vi "Teleop.vi"(10 "Match Info":T1={"Autonomous Elapsed Seconds"=0.0, "TeleOp Elapsed Seconds"=0.0, "Disabled Elapsed Seconds"=0.0, "Visited Autonomous"=FALSE, "Visited TeleOp"=FALSE, "Visited Disabled"=FALSE, "Autonomous Settings"={"Autonomous Style"=enum."Independent", "VI Refnum"=refnum}}, 11 "Call Context":T2) -> ()   [LabVIEW 2016]
doc: "This VI is called for each TeleOp packet received from the DS where the robot is not disabled. It is often used to read from the joysticks and update I/O or to update setpoints for timed control loops. It should complete and return within 20 milliseconds or it may miss DS packets."
uses:
  <vilib>/Rock Robotics/WPI/DriverStation/WPI_DriverStationDerivedRobotMode.ctl
  <vilib>/Rock Robotics/WPI/DriverStation/WPI_DriverStationMatch Info.ctl
  <vilib>/Rock Robotics/WPI/Solenoid/WPI_SolenoidValue.ctl
  Robot Global Data.vi
  <vilib>/Rock Robotics/WPI/Utilities/WPI_GetSetVariantRefNum.vi
  <vilib>/Rock Robotics/WPI/Solenoid/Deprecated/WPI_SolenoidSetBool.vi
  <vilib>/Rock Robotics/Network Tables/NT Write Number.vi
  <vilib>/Rock Robotics/Network Tables/NT Write Boolean.vi
  <vilib>/Rock Robotics/WPI/Solenoid/WPI_SolenoidSetEnum.vi
  navX Library v2/navX Library v2.lvlib
panel:
  out "Shooter Values":dbl[](graph)
  out "Shooter Values":cluster{dbl, "Sensor Velocity":dbl, dbl}(graph)
  out "Temperature":dbl(graph)
  in  "Ramp Rate":dbl format="%#_13g"
  in  "I Zone":dbl=3000.0 format="%#_13g"
  in  "F":dbl=0.005212 format="%#_13g"
  in  "D":dbl format="%#_13g"
  in  "I":dbl=0.001 format="%#_13g"
  out "Shooter 2":cluster{"Sensor Velocity":dbl, dbl, dbl}(graph)
  in  "ShooterRPM":dbl=-22000.0
  in  "P":dbl=0.2 format="%#_13g"
  in  "MOE":dbl=25.0 format="%#_13g"
  in  "Center":dbl=180.0 format="%#_13g"
  out "out left":dbl
  out "out right":dbl
  in  "Speed":dbl=0.45 format="%#_13g"
  out "Out Left":dbl(graph)
  out "Out Right":dbl(graph)
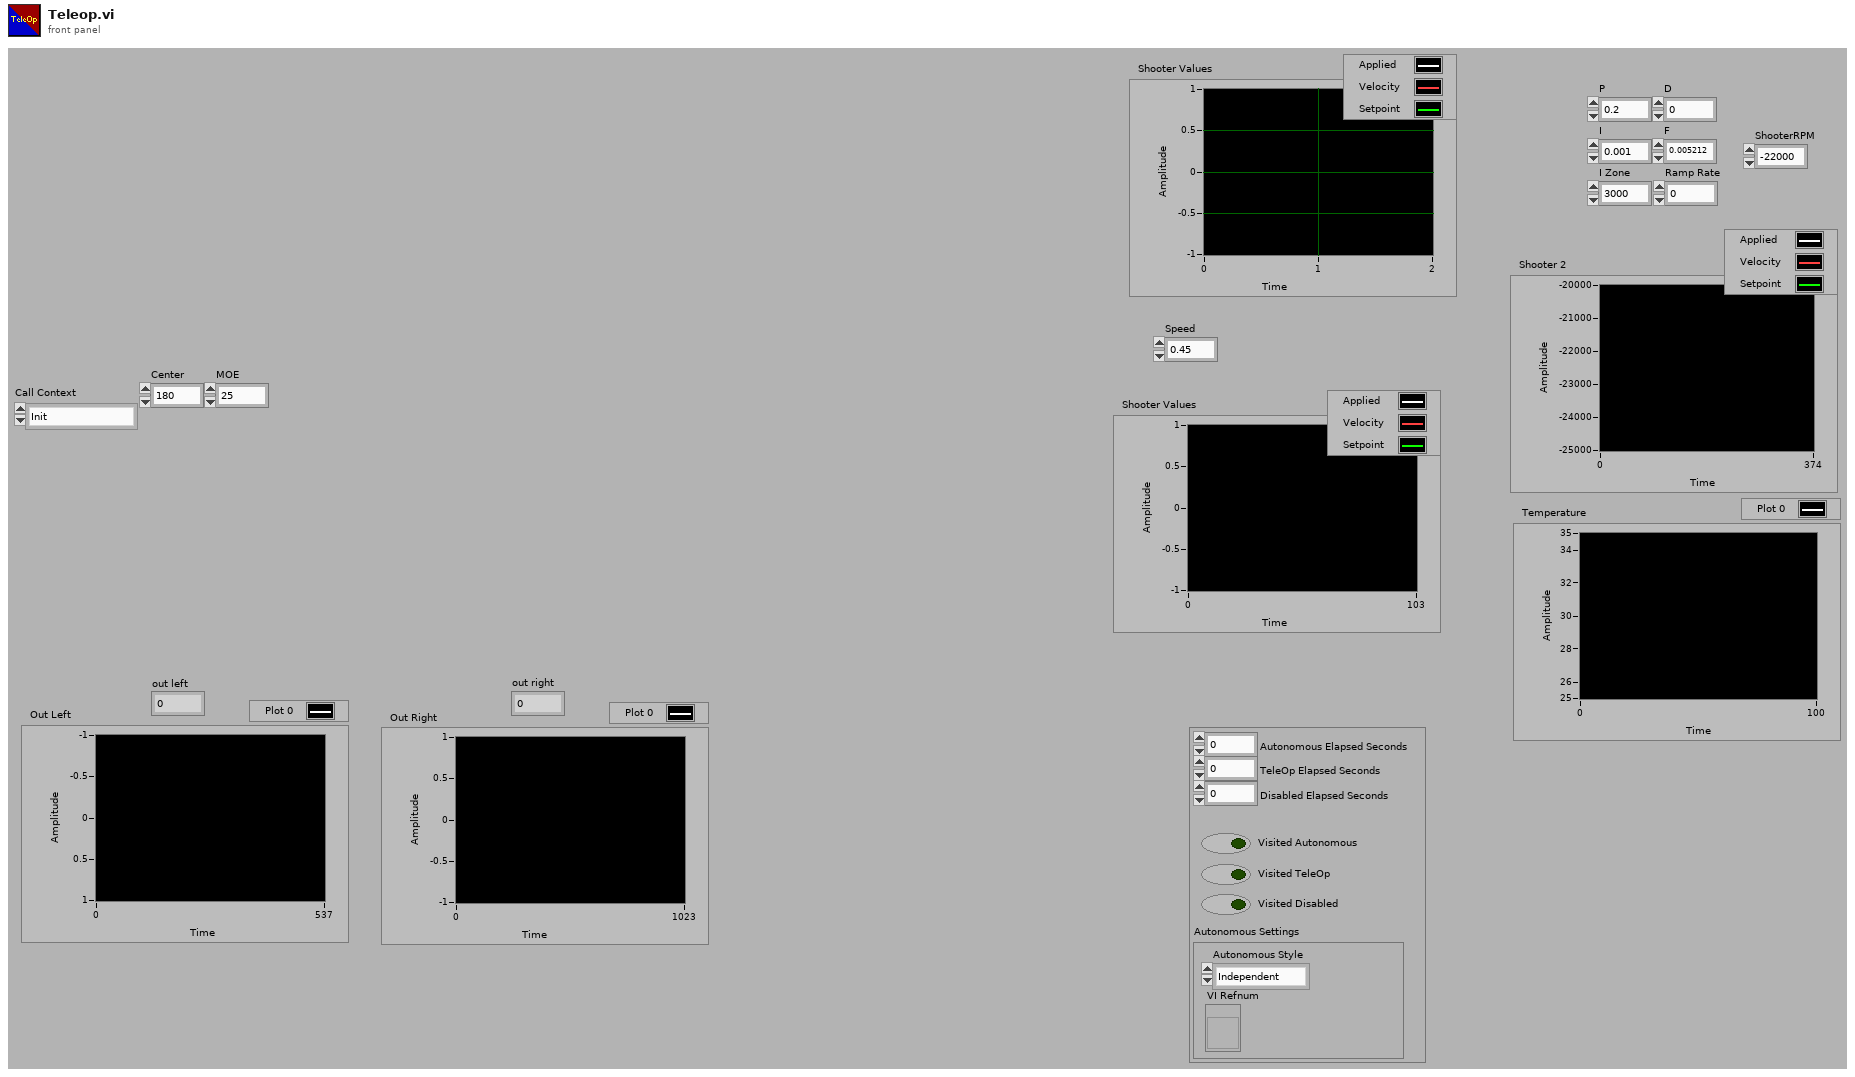
[diagram p1: front panel]
types:
  T1 = typedef "WPI_DriverStationMatch Info.ctl" = cluster{"Autonomous Elapsed Seconds":dbl, "TeleOp Elapsed Seconds":dbl, "Disabled Elapsed Seconds":dbl, "Visited Autonomous":bool, "Visited TeleOp":bool, "Visited Disabled":bool, "Autonomous Settings":cluster{"Autonomous Style":enum16{"Iterative", "Independent"}, "VI Refnum":refnum<vi>}}
  T2 = typedef "WPI_DriverStationDerivedRobotMode.ctl" = enum16{"Init", "Execute", "Stop"}
  T3 = typedef "WPI_SolenoidValue.ctl" = enum16{"Off", "On", "Forward", "Reverse"}
  T4 = typedef "WPI_SolenoidDevRef.ctl" = cluster{"DevStatus":errorcluster, "Pneumatics Control Module":u8, "Forward Solenoid Channel":T5, "Reverse Solenoid Channel":T5}
  T5 = typedef "WPI_SolenoidChannel.ctl" = enum8{"Solenoid 0", "Solenoid 1", "Solenoid 2", "Solenoid 3", "Solenoid 4", "Solenoid 5", "Solenoid 6", "Solenoid 7", "Invalid"}
  T6 = typedef "WPI_JoystickDevRef.ctl" = cluster{"Device":T7}
  T7 = typedef "WPI_JoystickDeviceEnum.ctl" = enum16{"USB 0", "USB 1", "USB 2", "USB 3", "USB 4", "USB 5"}
  T8 = cluster{"Buttons[0]":bool, "Buttons[1]":bool, "Buttons[2]":bool, "Buttons[3]":bool, "Buttons[4]":bool, "Buttons[5]":bool, "Buttons[6]":bool, "Buttons[7]":bool, "Buttons[8]":bool}
  T9 = cluster{"Axes[0]":dbl, "Axes[1]":dbl, "Axes[2]":dbl, "Axes[3]":dbl, "Axes[4]":dbl, "Axes[5]":dbl, "Axes[6]":dbl, "Axes[7]":dbl, "Axes[8]":dbl}
  T10 = typedef "navX Library v2.lvlib/Z900_navX_DeviceTypeDef.ctl" = cluster{"Interface":cluster{"Protocol":T11, "Update Rate (4Hz-100Hz)":u8, "navX Open TypeDef":variant}, "Notify Packet":refnum<notifier>, "Loop VI Refnum":refnum<vi>, "Ready to Close Occurrence Refnum":refnum<k4>}
  T11 = typedef "navX Library v2.lvlib/Z900_navX_ProtocolTypeDef.ctl" = enum16{"SERIAL", "I2C", "SPI"}
  T12 = cluster{"Velocity X":dbl, "Velocity Y":dbl, "Velocity Z":dbl, "Displacement X":dbl, "Displacement Y":dbl, "Displacement Z":dbl}
  T13 = cluster{"LinearAcceleration X":dbl, "LinearAcceleration Y":dbl, "LinearAcceleration Z":dbl}
  T14 = cluster{"Yaw":dbl, "Roll":dbl, "Pitch":dbl, "Heading":dbl, "Fused Heading":dbl}
  T15 = typedef "WPI_MotorControlDeviceRef.ctl" = cluster{"DeviceStatus":errorcluster, "Type":T16, "PWM":cluster{"PWM Channel":T17, "DeadBand":T18}, "CAN":cluster{"Device Number":u8, "SetOutput VI Ref":variant, "GetOutput VI Ref":variant, "Enable VI Ref":variant, "Disable VI Ref":variant, "Data":variant}, "Invert":bool}
  T16 = typedef "WPI_MotorControlType.ctl" = enum16{"PWM", "CAN"}
  T17 = typedef "FPGA_DIOPWMChannel.ctl" = enum8{"PWM 0", "PWM 1", "PWM 2", "PWM 3", "PWM 4", "PWM 5", "PWM 6", "PWM 7", "PWM 8", "PWM 9", "PWM MXP 0", "PWM MXP 1", "PWM MXP 2", "PWM MXP 3", "PWM MXP 4", "PWM MXP 5", "PWM MXP 6", "PWM MXP 7", "PWM MXP 8", "PWM MXP 9", "Invalid"}
  T18 = typedef "WPI_PWMDeadband.ctl" = cluster{"Name":string, "maxPositivePwm":i32, "minPositivePwm":i32, "centerPwm":i32, "maxNegativePwm":i32, "minNegativePwm":i32, "angularRange":u16}
  T19 = typedef "WPI_CANTalonSRX_GlobalStatus.ctl" = cluster{"Applied Throttle":dbl, "Module Enabled":bool, "CAN Error":errorcluster, "Closed Loop Error":dbl, "Forward Limit Switch Closed":bool, "Reverse Limit Switch Closed":bool, "Sensor Position":dbl, "Sensor Velocity":dbl, "Current":dbl, "Sticky Fault - Over Temp":bool, "Sticky Fault - Under Voltage":bool, "Sticky Fault - Forward Limit":bool, "Sticky Fault - Reverse Limit":bool, "Sticky Fault - Forward Soft Limit":bool, "Sticky Fault - Reverse Soft Limit":bool, "Brake is Enabled":bool, "Encoder Position":dbl, "Encoder Velocity":dbl, "Encoder Index Count":dbl, "Encoder A Pin State":bool, "Encoder B Pin State":bool, "Encoder Index Pin State":bool, "Analog In":dbl, "Analog In Velocity":dbl, "Temperature (C)":dbl, "Battery Voltage":dbl, "Control 5 Is Supported":bool, "Current Profile Slot Select":dbl, "Pos Div 8":bool, "Vel Div 4":bool, "Pulse Width Position":i32, "Pulse Width Velocity":i32, "Pulse Width Rise To Rise (us)":i32, "Pulse Width Rise To Fall (us)":i32, "Mot Prof Active Is Under Run":bool, "Mot Prof Active Has Under Run":bool, "Mot Prof Active Is Last":bool, "Mot Prof Active Velocity Only":bool, "Mot Prof Active Is Valid":bool, "Mot Prof Buffer Is Full":bool, "Mot Prof Active Profile Slot Select":i32, "Mot Prof NextID":i32, "Mot Prof Count":i32, "Mot Prof Active Velocity":dbl, "Mot Prof Active Position":dbl, "Mot Prof Output Enable":i32}
  T20 = typedef "WPI_RobotDriveDevRef.ctl" = cluster{"DevStatus":errorcluster, "Motors[]":T15[], "Square Inputs":bool, "Max Output":dbl}
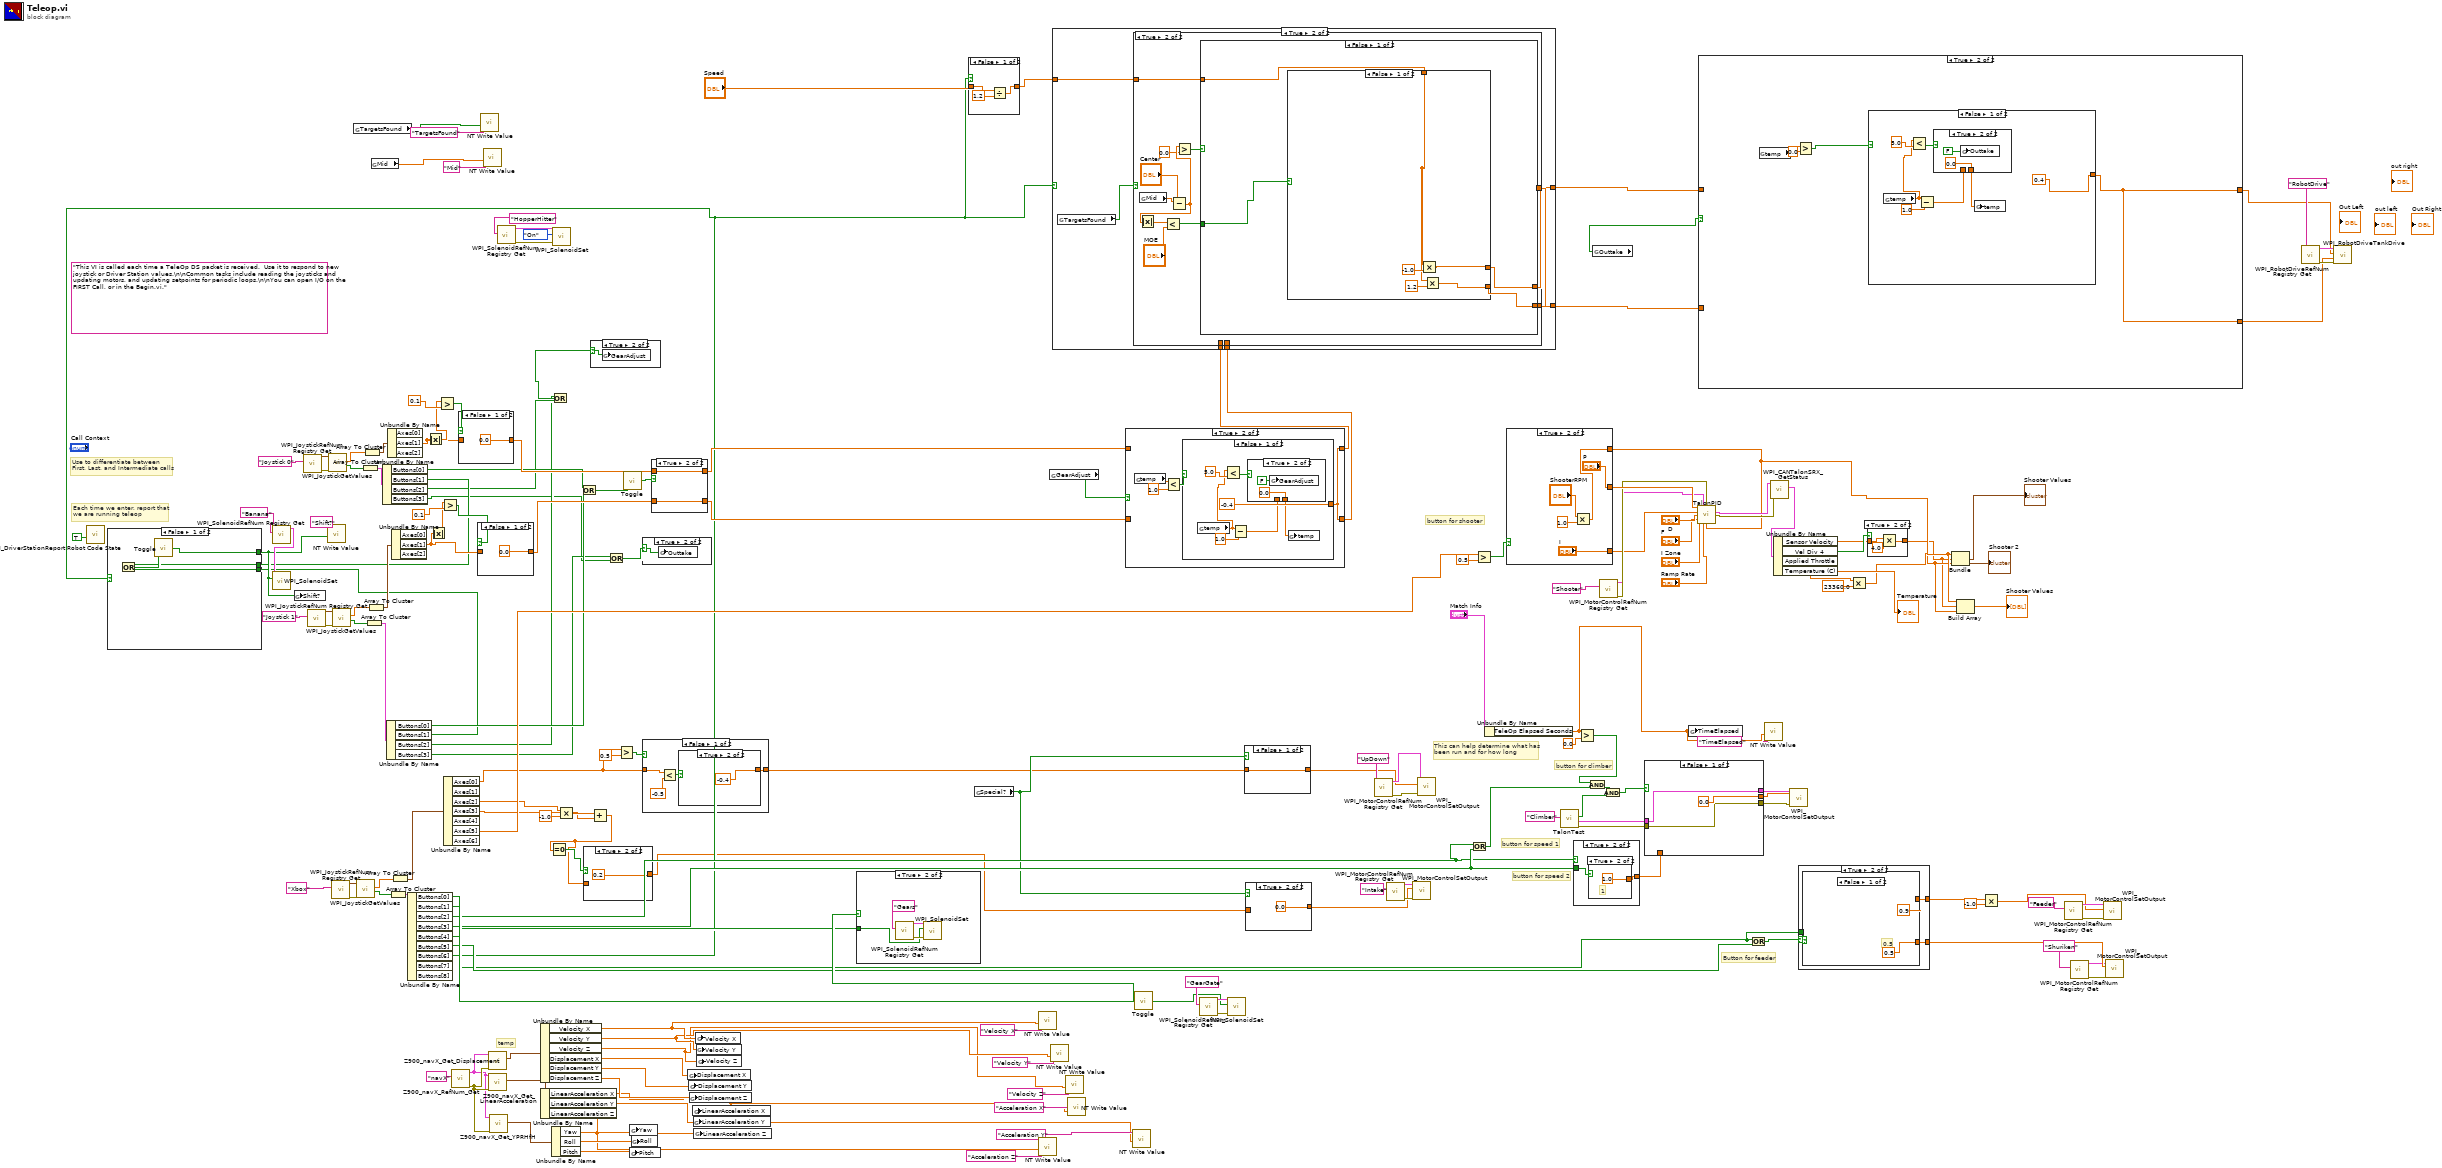
[diagram p0: block diagram]
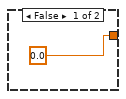
[diagram p3: hidden frame]
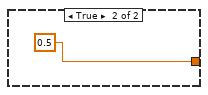
[diagram p4: hidden frame]
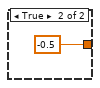
[diagram p6: hidden frame]
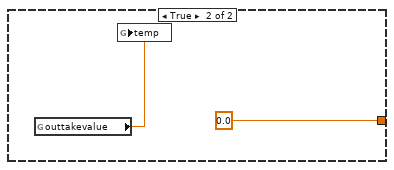
[diagram p9: hidden frame]
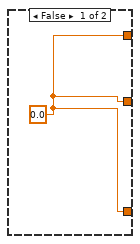
[diagram p12: hidden frame]
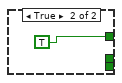
[diagram p13: hidden frame]
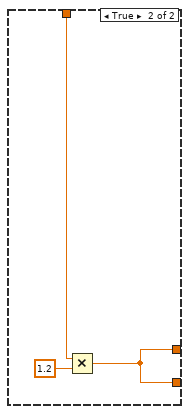
[diagram p17: hidden frame]
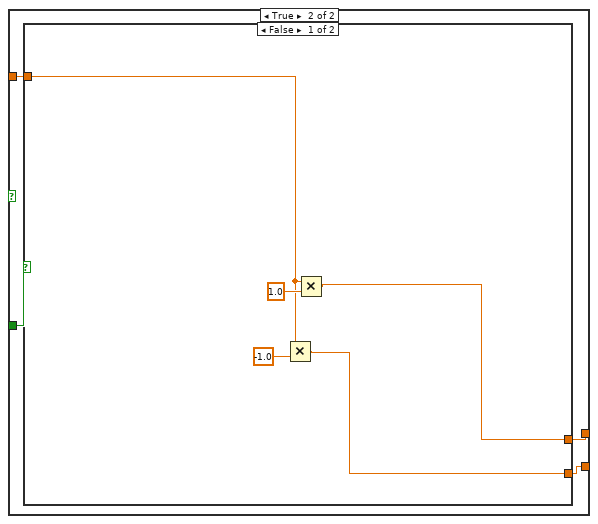
[diagram p18: hidden frame]
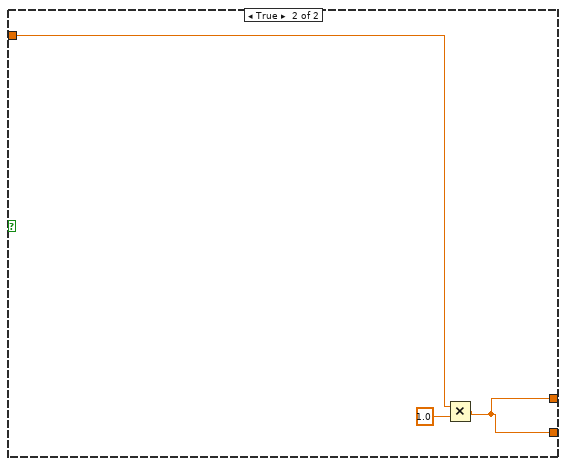
[diagram p19: hidden frame]
diagram:
  (unwired) "This VI is called each time a TeleOp DS packet is received.  Use it to respond to new joystick or Driver Station values.\n\nCommon tasks include reading the joysticks and updating motors, and updating setpoints for periodic loops.\n\nYou can open I/O on the FIRST Call, or in the Begin.vi."
  # "button for shooter"
  # "temp"
  # "Button for feeder"
  # "button for speed 2"
  # "button for speed 1"
  # "button for climber"
  # "Each time we enter, report that\nwe are running teleop"
  # "Use to differentiate between\nFirst, Last, and Intermediate calls"
  # "This can help determine what has\nbeen run and for how long"
  n1 = call <vilib>:"WPI_DriverStationReport Robot Code State.vi"("TeleOp"=TRUE ("Autonomous")) -> ()  [unwired: 10 in, 1 out]
  n2 = call <vilib>:"WPI_SolenoidRefNum Registry Get.vi"("refnum name"="Banana") -> ("SolenoidDevRef"=w94:T4)  [unwired: 9 in, 1 out]
  n3 = call <vilib>:"WPI_JoystickRefNum Registry Get.vi"("refnum name"="Joystick 0") -> ("error out"=w177:errorcluster, "JoystickDevRef"=w176:T6)  [unwired: 9 in]
  n4 = call <vilib>:"WPI_JoystickRefNum Registry Get.vi"("refnum name"="Joystick 1") -> ("error out"=w169:errorcluster, "JoystickDevRef"=w168:T6)  [unwired: 9 in]
  n5 = call <vilib>:"WPI_JoystickGetValues.vi"("error in (no error)"=w177, "JoystickDevRef"=w176) -> ("Buttons"=w173:bool[], "Axes"=w174:dbl[])  [unwired: 5 in, 3 out]
  n6 = call <vilib>:"WPI_JoystickRefNum Registry Get.vi"("refnum name"="Xbox") -> ("error out"=w144:errorcluster, "JoystickDevRef"=w143:T6)  [unwired: 9 in]
  n7 = call <vilib>:"WPI_JoystickGetValues.vi"("error in (no error)"=w169, "JoystickDevRef"=w168) -> ("Buttons"=w165:bool[], "Axes"=w166:dbl[])  [unwired: 5 in, 3 out]
  n8 = global read "Robot Global Data.vi" "TargetsFound"() -> (w98:bool)
  n9 = call <vilib>:"WPI_JoystickGetValues.vi"("error in (no error)"=w144, "JoystickDevRef"=w143) -> ("Buttons"=w140:bool[], "Axes"=w141:dbl[])  [unwired: 5 in, 3 out]
  n10 = Array To Cluster(array=w173) -> (cluster=w171:T8)
  n11 = Array To Cluster(array=w174) -> (cluster=w172:T9)
  n12 = Array To Cluster(array=w165) -> (cluster=w163:T8)
  n13 = Array To Cluster(array=w166) -> (cluster=w164:T9)
  n14 = global read "Robot Global Data.vi" "Mid"() -> (w96:dbl)
  n15 = Unbundle By Name(w171) -> ("Buttons[0]"=w36:bool, "Buttons[1]"=w32:bool, "Buttons[2]"=w31:bool, "Buttons[3]"=w19:bool)
  n16 = Unbundle By Name(w163) -> ("Buttons[0]"=w35:bool, "Buttons[1]"=w33:bool, "Buttons[2]"=w30:bool, "Buttons[3]"=w20:bool)
  n17 = Unbundle By Name(w172) -> ("Axes[1]"=w158:dbl)  [unwired: 2 out]
  n18 = Array To Cluster(array=w140) -> (cluster=w138:T8)
  n19 = Unbundle By Name(w164) -> ("Axes[1]"=w160:dbl)  [unwired: 2 out]
  n20 = Array To Cluster(array=w141) -> (cluster=w139:T9)
  n21 = Unbundle By Name(w138) -> ("Buttons[0]"=w137:bool, "Buttons[1]"=w136:bool, "Buttons[2]"=w37:bool, "Buttons[3]"=w135:bool, "Buttons[4]"=w132:bool, "Buttons[5]"=w133:bool, "Buttons[6]"=w29:bool)  [unwired: 2 out]
  n22 = case shown="False" w29 {
    tunnel: w33 -> [w181 _]
    tunnel: w32 -> [w180 _]
    tunnel: [w179 TRUE] -> w92
    frame False {
      n23 = Or(x=w180, y=w181) -> (x .or. y?=w182:bool)
      n24 = call "Toggle.vi"("Input"=w182) -> ("Output"=w179:bool)
    }
    frame True {
    }
  }
  n25 = call-poly <vilib>:"WPI_SolenoidSet.vi"("Value"=w92, "SolenoidDevRef"=w94) -> ()  [unwired: 8 in, 2 out]
  n26 = global write "Robot Global Data.vi" "Shift?"(w92) -> ()
  n27 = call-poly <vilib>:"NT Write Value.vi"("Boolean"=w92, "Name"="Shift?") -> ()  [unwired: 9 in, 1 out]
  n28 = Absolute Value(x=w158) -> (abs(x)=w159:dbl)
  n29 = Absolute Value(x=w160) -> (abs(x)=w161:dbl)
  n30 = Greater?(x=w159, y=0.1 ("x")) -> (0:w110:bool)
  n31 = Greater?(x=w161, y=0.1 ("x")) -> (0:w109:bool)
  n32 = Unbundle By Name(w139) -> ("Axes[0]"=w5:dbl, "Axes[2]"=w28:dbl, "Axes[3]"=w25:dbl, "Axes[5]"=w74:dbl)  [unwired: 3 out]
  n33 = call "Z900_navX_RefNum_Get.vi"("refnum name"="navX") -> ("error out"=w61:errorcluster, "navX Device"=w60:T10)  [unwired: 9 in]
  n34 = case shown="False" w110 {
    tunnel: w158 -> [_ w185]
    tunnel: [0.0 w185] -> w107
    frame False {
    }
    frame True {
    }
  }
  n35 = case shown="False" w109 {
    tunnel: w160 -> [_ w187]
    tunnel: [0.0 w187] -> w108
    frame False {
    }
    frame True {
    }
  }
  n36 = call-poly <vilib>:"NT Write Value.vi"("Boolean"=w98, "Name"="TargetsFound") -> ()  [unwired: 9 in, 1 out]
  n37 = call-poly <vilib>:"NT Write Value.vi"("Numeric"=w96, "Name"="Mid") -> ()  [unwired: 9 in, 1 out]
  n38 = call "Z900_navX_Get_Displacement.vi"("error in (no error)"=w61, "navX Device"=w60) -> ("Displacement"=w57:T12)  [unwired: 6 in, 3 out]
  n39 = call "Z900_navX_Get_LinearAcceleration.vi"("error in (no error)"=w61, "navX Device"=w60) -> ("Linear Acceleration"=w58:T13)  [unwired: 6 in, 3 out]
  n40 = call "Z900_navX_Get_YPRHfH.vi"("error in (no error)"=w61, "navX Device"=w60) -> ("YRPHfH"=w59:T14)  [unwired: 6 in, 3 out]
  n41 = call <vilib>:"WPI_SolenoidRefNum Registry Get.vi"("refnum name"="HopperHitter") -> ("error out"=w64:errorcluster, "SolenoidDevRef"=w65:T4)  [unwired: 9 in]
  n42 = Unbundle By Name(w57) -> ("Velocity X"=w45:dbl, "Velocity Y"=w44:dbl, "Velocity Z"=w43:dbl, "Displacement X"=w56:dbl, "Displacement Y"=w55:dbl, "Displacement Z"=w54:dbl)
  n43 = Unbundle By Name(w58) -> ("LinearAcceleration X"=w42:dbl, "LinearAcceleration Y"=w39:dbl, "LinearAcceleration Z"=w41:dbl)
  n44 = Or(x=w30, y=w31) -> (x .or. y?=w116:bool)
  n45 = Unbundle By Name(w59) -> ("Yaw"=w53:dbl, "Roll"=w52:dbl, "Pitch"=w51:dbl)
  n46 = call-poly <vilib>:"WPI_SolenoidSet.vi"("error in (no error)"=w64, "Value"=WPI_SolenoidValue."On", "SolenoidDevRef"=w65) -> ()  [unwired: 7 in, 2 out]
  n47 = Multiply(x=w28, y=-1.0) -> (x*y=w26:dbl)
  n48 = Or(x=w36, y=w35) -> (x .or. y?=w34:bool)
  n49 = case shown="True" w116 {
    selector: w116 -> [_ w188]
    frame False {
    }
    frame True {
      n50 = global write "Robot Global Data.vi" "GearAdjust"(w188) -> ()
    }
  }
  n51 = Add(x=w26, y=w25) -> (x+y=w2:dbl)
  n52 = Equal To 0?(x=w2) -> (x = 0?=w3:bool)
  n53 = case shown="True" w3 {
    tunnel: w2 -> [w189 _]
    tunnel: [w189 0.2] -> w1
    frame False {
    }
    frame True {
    }
  }
  n54 = Or(x=w20, y=w19) -> (x .or. y?=w21:bool)
  n55 = Greater?(x=w5, y=0.5) -> (0:w6:bool)
  n56 = call "Toggle.vi"("Input"=w34) -> ("Output"=w104:bool)
  n57 = global write "Robot Global Data.vi" "Pitch"(w51) -> ()
  n58 = global write "Robot Global Data.vi" "Yaw"(w53) -> ()
  n59 = global write "Robot Global Data.vi" "Roll"(w52) -> ()
  n60 = case shown="True" w21 {
    selector: w21 -> [_ w191]
    frame False {
    }
    frame True {
      n61 = global write "Robot Global Data.vi" "Outtake"(w191) -> ()
    }
  }
  n62 = case shown="False" w6 {
    tunnel: w5 -> [w194 _]
    tunnel: [w192 0.5] -> w4
    frame False {
      n63 = Less?(x=w194, y=-0.5) -> (x < y?=w195:bool)
      n64 = case shown="True" w195 {
        tunnel: [0.0 -0.4] -> w192
        frame False {
        }
        frame True {
        }
      }
    }
    frame True {
    }
  }
  n65 = case shown="True" w104 {
    tunnel: w107 -> [w200 w205]
    tunnel: w108 -> [w199 w204]
    tunnel: [w203 w205] -> w106
    tunnel: [w202 w204] -> w105
    frame False {
      w201 = -1.0
      n66 = Multiply(x=w201, y=w200) -> (x*y=w202:dbl)
      n67 = Multiply(x=w199, y=w201) -> (x*y=w203:dbl)
    }
    frame True {
    }
  }
  n68 = global write "Robot Global Data.vi" "Displacement X"(w56) -> ()
  n69 = global write "Robot Global Data.vi" "Displacement Y"(w55) -> ()
  n70 = global write "Robot Global Data.vi" "Displacement Z"(w54) -> ()
  n71 = global write "Robot Global Data.vi" "LinearAcceleration X"(w42) -> ()
  n72 = global write "Robot Global Data.vi" "LinearAcceleration Y"(w39) -> ()
  n73 = global write "Robot Global Data.vi" "LinearAcceleration Z"(w41) -> ()
  n74 = global write "Robot Global Data.vi" "Velocity X"(w45) -> ()
  n75 = global write "Robot Global Data.vi" "Velocity Y"(w44) -> ()
  n76 = global write "Robot Global Data.vi" "Velocity Z"(w43) -> ()
  n77 = case shown="False" w29 {
    tunnel: [w208 w209] -> w102
    tunnel: "Speed" -> [w207 w209]
    frame False {
      n78 = Divide(x=w207, y=1.2) -> (x/y=w208:dbl)
    }
    frame True {
    }
  }
  n79 = global read "Robot Global Data.vi" "Special?"() -> (w12:bool)
  n80 = call-poly <vilib>:"NT Write Value.vi"("Numeric"=w45, "Name"="Velocity X") -> ()  [unwired: 9 in, 1 out]
  n81 = call-poly <vilib>:"NT Write Value.vi"("Numeric"=w41, "Name"="Acceleration Z") -> ()  [unwired: 9 in, 1 out]
  n82 = global read "Robot Global Data.vi" "GearAdjust"() -> (w117:bool)
  n83 = call-poly <vilib>:"NT Write Value.vi"("Numeric"=w44, "Name"="Velocity Y") -> ()  [unwired: 9 in, 1 out]
  n84 = call-poly <vilib>:"NT Write Value.vi"("Numeric"=w43, "Name"="Velocity Z") -> ()  [unwired: 9 in, 1 out]
  n85 = call-poly <vilib>:"NT Write Value.vi"("Numeric"=w42, "Name"="Acceleration X") -> ()  [unwired: 9 in, 1 out]
  n86 = case shown="True" w117 {
    tunnel: w106 -> [w211 _]
    tunnel: w105 -> [w210 _]
    tunnel: [w211 w212] -> w112
    tunnel: [w210 w212] -> w111
    frame False {
    }
    frame True {
      n87 = global read "Robot Global Data.vi" "temp"() -> (w215:dbl)
      n88 = Less?(x=w215, y=1.0) -> (x < y?=w213:bool)
      n89 = case shown="False" w213 {
        tunnel: [-0.4 0.0] -> w212
        frame False {
          n90 = global read "Robot Global Data.vi" "temp"() -> (w218:dbl)
          n91 = Less?(x=w218, y=5.0 ("x")) -> (x < y?=w219:bool)
          n92 = Subtract(x=w218, y=1.0) -> (x-y=w216:dbl)
          n93 = case shown="True" w219 {
            tunnel: [w223 0.0] -> w217
            tunnel: w216 -> [w223 _]
            frame False {
            }
            frame True {
              n94 = global write "Robot Global Data.vi" "GearAdjust"(FALSE) -> ()
            }
          }
          n95 = global write "Robot Global Data.vi" "temp"(w217) -> ()
        }
        frame True {
          n96 = global read "Robot Global Data.vi" "GearAdjustValue"() -> (w227:dbl)
          n97 = global write "Robot Global Data.vi" "temp"(w227) -> ()
        }
      }
    }
  }
  n98 = case shown="True" w29 {
    tunnel: w112 -> [w229 w235]
    tunnel: w111 -> [w228 w234]
    tunnel: [w229 w230] -> w18
    tunnel: [w228 w231] -> w17
    tunnel: w102 -> [_ w232]
    frame False {
    }
    frame True {
      n99 = global read "Robot Global Data.vi" "TargetsFound"() -> (w233:bool)
      n100 = case shown="True" w233 {
        tunnel: w235 -> [w236 _]
        tunnel: w234 -> [w237 _]
        tunnel: [w236 w243] -> w230
        tunnel: [w237 w242] -> w231
        tunnel: w232 -> [_ w238]
        frame False {
        }
        frame True {
          n101 = global read "Robot Global Data.vi" "Mid"() -> (w248:dbl)
          n102 = Subtract(x=w248, y="Center") -> (x-y=w240:dbl)
          n103 = Absolute Value(x=w240) -> (abs(x)=w246:dbl)
          n104 = Less?(x=w246, y="MOE") -> (x < y?=w244:bool)
          n105 = Greater?(x=w240, y=0.0) -> (0:w241:bool)
          n106 = case shown="False" w241 {
            tunnel: w244 -> [w252 w264]
            tunnel: [w249 w262] -> w243
            tunnel: [w250 w263] -> w242
            tunnel: w238 -> [w251 w261]
            frame False {
              n107 = case shown="False" w252 {
                tunnel: [w257 w260] -> w250
                tunnel: [w255 w260] -> w249
                tunnel: w251 -> [w253 w258]
                frame False {
                  n108 = Multiply(x=w253, y=-1.0) -> (x*y=w257:dbl)
                  n109 = Multiply(x=w253, y=1.2) -> (x*y=w255:dbl)
                }
                frame True {
                  n110 = Multiply(x=w258, y=1.2) -> (x*y=w260:dbl)
                }
              }
            }
            frame True {
              n111 = case shown="False" w264 {
                tunnel: [w269 w272] -> w263
                tunnel: [w267 w272] -> w262
                tunnel: w261 -> [w265 w270]
                frame False {
                  n112 = Multiply(x=w265, y=-1.0) -> (x*y=w267:dbl)
                  n113 = Multiply(x=w265, y=1.0) -> (x*y=w269:dbl)
                }
                frame True {
                  n114 = Multiply(x=w270, y=1.0) -> (x*y=w272:dbl)
                }
              }
            }
          }
        }
      }
    }
  }
  n115 = call-poly <vilib>:"NT Write Value.vi"("Numeric"=w39, "Name"="Acceleration Y") -> ()  [unwired: 9 in, 1 out]
  n116 = call "Toggle.vi"("Input"=w137) -> ("Output"=w145:bool)
  n117 = case shown="True" w145 {
    tunnel: w136 -> [_ w273]
    frame False {
    }
    frame True {
      n118 = call <vilib>:"WPI_SolenoidRefNum Registry Get.vi"("refnum name"="Gears") -> ("error out"=w276:errorcluster, "SolenoidDevRef"=w275:T4)  [unwired: 9 in]
      n119 = call-poly <vilib>:"WPI_SolenoidSet.vi"("error in (no error)"=w276, "Value"=w273, "SolenoidDevRef"=w275) -> ()  [unwired: 7 in, 2 out]
    }
  }
  n120 = call <vilib>:"WPI_SolenoidRefNum Registry Get.vi"("refnum name"="GearGate") -> ("error out"=w148:errorcluster, "SolenoidDevRef"=w147:T4)  [unwired: 9 in]
  n121 = call-poly <vilib>:"WPI_SolenoidSet.vi"("error in (no error)"=w148, "Value"=w145, "SolenoidDevRef"=w147) -> ()  [unwired: 7 in, 2 out]
  n122 = case shown="False" w12 {
    tunnel: [w277 -0.5] -> w13
    tunnel: w4 -> [w277 _]
    frame False {
    }
    frame True {
    }
  }
  n123 = case shown="True" w12 {
    tunnel: [w279 0.0] -> w8
    tunnel: w1 -> [w279 _]
    frame False {
    }
    frame True {
    }
  }
  n124 = call <vilib>:"WPI_MotorControlRefNum Registry Get.vi"("refnum name"="UpDown") -> ("error out"=w24:errorcluster, "MotorControlDevRef"=w23:T15)  [unwired: 9 in]
  n125 = call <vilib>:"WPI_MotorControlRefNum Registry Get.vi"("refnum name"="Intake") -> ("error out"=w10:errorcluster, "MotorControlDevRef"=w11:T15)  [unwired: 9 in]
  n126 = call <vilib>:"WPI_MotorControlSetOutput.vi"("error in (no error)"=w10, "Output"=w8, "MotorControlDevRef"=w11) -> ()  [unwired: 6 in, 3 out]
  n127 = call <vilib>:"WPI_MotorControlSetOutput.vi"("error in (no error)"=w24, "Output"=w13, "MotorControlDevRef"=w23) -> ()  [unwired: 6 in, 3 out]
  n128 = Or(x=w37, y=w135) -> (x .or. y?=w134:bool)
  n129 = Greater?(x=w74, y=0.5) -> (0:w75:bool)
  n130 = Unbundle By Name("Match Info") -> ("TeleOp Elapsed Seconds"=w101:dbl)
  n131 = case shown="True" w75 {
    tunnel: [w281 w284] -> w70
    tunnel: [w281 "P"] -> w80
    tunnel: [w281 "I"] -> w67
    frame False {
      w281 = 0.0
    }
    frame True {
      n132 = Multiply(x="ShooterRPM", y=1.0) -> (x*y=w284:dbl)
    }
  }
  n133 = call "TalonTest.vi"("Name"="Climber") -> ("Output"=w155:bool, "Ref"=w151:T15, "error out"=w150:errorcluster)  [unwired: 7 in]
  n134 = case shown="True" w37 {
    tunnel: [w288 w292] -> w149
    tunnel: w135 -> [w287 w291]
    frame False {
      n135 = case shown="False" w287 {
        tunnel: [0.0 0.25] -> w288
        frame False {
        }
        frame True {
          # "0.25"
        }
      }
    }
    frame True {
      n136 = case shown="True" w291 {
        tunnel: [0.75 1.0] -> w292
        frame False {
          # "0.75"
        }
        frame True {
          # "1"
        }
      }
    }
  }
  n137 = Greater?(x=w101, y=0.0) -> (0:w153:bool)
  n138 = And(x=w153, y=w134) -> (x .and. y?=w156:bool)
  n139 = global read "Robot Global Data.vi" "Outtake"() -> (w16:bool)
  n140 = call <vilib>:"WPI_MotorControlRefNum Registry Get.vi"("refnum name"="Shooter" ("Name")) -> ("error out"=w78:errorcluster, "MotorControlDevRef"=w77:T15)  [unwired: 9 in]
  n141 = And(x=w156, y=w155) -> (x .and. y?=w152:bool)
  n142 = case shown="False" w152 {
    tunnel: w151 -> [w296 w300]
    tunnel: w150 -> [w295 w298]
    tunnel: w149 -> [_ w299]
    tunnel: [w296 w300] -> w129
    tunnel: [0.0 w299] -> w130
    tunnel: [w295 w298] -> w128
    frame False {
    }
    frame True {
    }
  }
  n143 = global write "Robot Global Data.vi" "TimeElapsed"(w101) -> ()
  n144 = call "TalonPID.vi"("P"=w80, "Ref In"=w77, "Error in"=w78, "I"=w67, "D"="D", "F"="F", "I Zone"="I Zone", "Ramp Rate"="Ramp Rate", "Output"=w70) -> ("Ref Out"=w82:T15, "error out"=w81:errorcluster)  [unwired: 5 in]
  n145 = case shown="True" w16 {
    tunnel: w18 -> [w301 _]
    tunnel: w17 -> [w302 _]
    tunnel: [w302 w304] -> w15
    tunnel: [w301 w304] -> w14
    frame False {
    }
    frame True {
      n146 = global read "Robot Global Data.vi" "temp"() -> (w306:dbl)
      n147 = Greater?(x=w306, y=0.0) -> (0:w303:bool)
      n148 = case shown="False" w303 {
        tunnel: [0.4 0.0] -> w304
        frame False {
          n149 = global read "Robot Global Data.vi" "temp"() -> (w310:dbl)
          n150 = Less?(x=w310, y=5.0 ("x")) -> (x < y?=w311:bool)
          n151 = Subtract(x=w310, y=1.0) -> (x-y=w308:dbl)
          n152 = case shown="True" w311 {
            tunnel: [w314 0.0] -> w309
            tunnel: w308 -> [w314 _]
            frame False {
            }
            frame True {
              n153 = global write "Robot Global Data.vi" "Outtake"(FALSE) -> ()
            }
          }
          n154 = global write "Robot Global Data.vi" "temp"(w309) -> ()
        }
        frame True {
          n155 = global read "Robot Global Data.vi" "outtakevalue"() -> (w317:dbl)
          n156 = global write "Robot Global Data.vi" "temp"(w317) -> ()
        }
      }
    }
  }
  n157 = Or(x=w132, y=w133) -> (x .or. y?=w131:bool)
  n158 = call-poly <vilib>:"NT Write Value.vi"("Numeric"=w101, "Name"="TimeElapsed") -> ()  [unwired: 9 in, 1 out]
  n159 = call <vilib>:"WPI_CANTalonSRX_GetStatus.vi"("error in (no error)"=w81, "CAN Talon SRX Ref"=w82) -> ("Talon SRX Status"=w91:T19)  [unwired: 7 in, 2 out]
  n160 = Unbundle By Name(w91) -> ("Sensor Velocity"=w89:dbl, "Vel Div 4"=w90:bool, "Applied Throttle"=w87:dbl, "Temperature (C)"=→"Temperature":dbl)
  n161 = call <vilib>:"WPI_MotorControlSetOutput.vi"("error in (no error)"=w128, "Output"=w130, "MotorControlDevRef"=w129) -> ()  [unwired: 6 in, 3 out]
  n162 = case shown="True" w131 {
    tunnel: w132 -> [_ w322]
    tunnel: [w319 w321] -> w120
    tunnel: [w319 w320] -> w127
    frame False {
      w319 = 0.0
    }
    frame True {
      n163 = case shown="False" w322 {
        tunnel: [0.9 ("Output") 0.9 ("Output")] -> w321
        tunnel: [0.5 ("Output") 0.5 ("Output")] -> w320
        frame False {
          # "0.5"
        }
        frame True {
          # "0.5"
        }
      }
    }
  }
  n164 = Multiply(x=w87, y=23360.0) -> (x*y=w71:dbl)
  n165 = case shown="True" w90 {
    tunnel: w89 -> [w327 w329]
    tunnel: [w327 w330] -> w69
    frame False {
    }
    frame True {
      n166 = Multiply(x=w329, y=4.0) -> (x*y=w330:dbl)
    }
  }
  n167 = Bundle(w71, "Sensor Velocity"=w69, w70) -> (→"Shooter 2" →"Shooter Values":cluster{dbl, "Sensor Velocity":dbl, dbl})  [unwired: 1 in]
  n168 = Build Array(w71, w69, w70) -> (→"Shooter Values":dbl[])
  n169 = Multiply(x=w120, y=-1.0) -> (x*y=w118:dbl)
  n170 = call <vilib>:"WPI_MotorControlRefNum Registry Get.vi"("refnum name"="Feeder") -> ("error out"=w121:errorcluster, "MotorControlDevRef"=w122:T15)  [unwired: 9 in]
  n171 = call <vilib>:"WPI_MotorControlRefNum Registry Get.vi"("refnum name"="Shuriken") -> ("error out"=w123:errorcluster, "MotorControlDevRef"=w124:T15)  [unwired: 9 in]
  n172 = call <vilib>:"WPI_MotorControlSetOutput.vi"("error in (no error)"=w121, "Output"=w118, "MotorControlDevRef"=w122) -> ()  [unwired: 6 in, 3 out]
  n173 = call <vilib>:"WPI_MotorControlSetOutput.vi"("error in (no error)"=w123, "Output"=w127, "MotorControlDevRef"=w124) -> ()  [unwired: 6 in, 3 out]
  n174 = call <vilib>:"WPI_RobotDriveRefNum Registry Get.vi"("refnum name"="RobotDrive") -> ("error out"=w115:errorcluster, "RobotDriveDevRef"=w114:T20)  [unwired: 9 in]
  n175 = call <vilib>:"WPI_RobotDriveTankDrive.vi"("error in (no error)"=w115, "Right axis value"=w15, "Left axis value"=w14, "RobotDriveDevRef"=w114) -> ()  [unwired: 5 in, 3 out]
